vi "Sec2Timestamp.vi"(7 "Input Selection":enum32{"Time (Double)", "Time (Time Stamp)"}(radio), 10 "Input Time (Time Stamp)":timestamp format="%<%H:%M:%S%3u\n%m/%d/%y>T", 11 "Input Time (Double)":dbl format="%<%H:%M:%S>t") -> (1 "date/time string":string, 2 "Time (Time Stamp)":timestamp format="%<%H:%M:%S%3u\n%m/%d/%y>T", 3 "Time (Double)":dbl format="%<%H:%M:%S%3u\n%m/%d/%Y>T")   [LabVIEW 2018]
panel:
  out "DST (Local)":bool
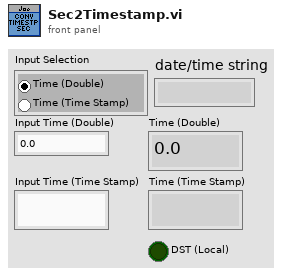
[diagram p1: front panel]
types:
  T1 = typedef "LVDateTimeRec.ctl" = cluster{"fractional second":dbl, "second":i32, "minute":i32, "hour":i32, "day of month":i32, "month":i32, "year":i32, "day of week":i32, "day of year":i32, "DST":i32}
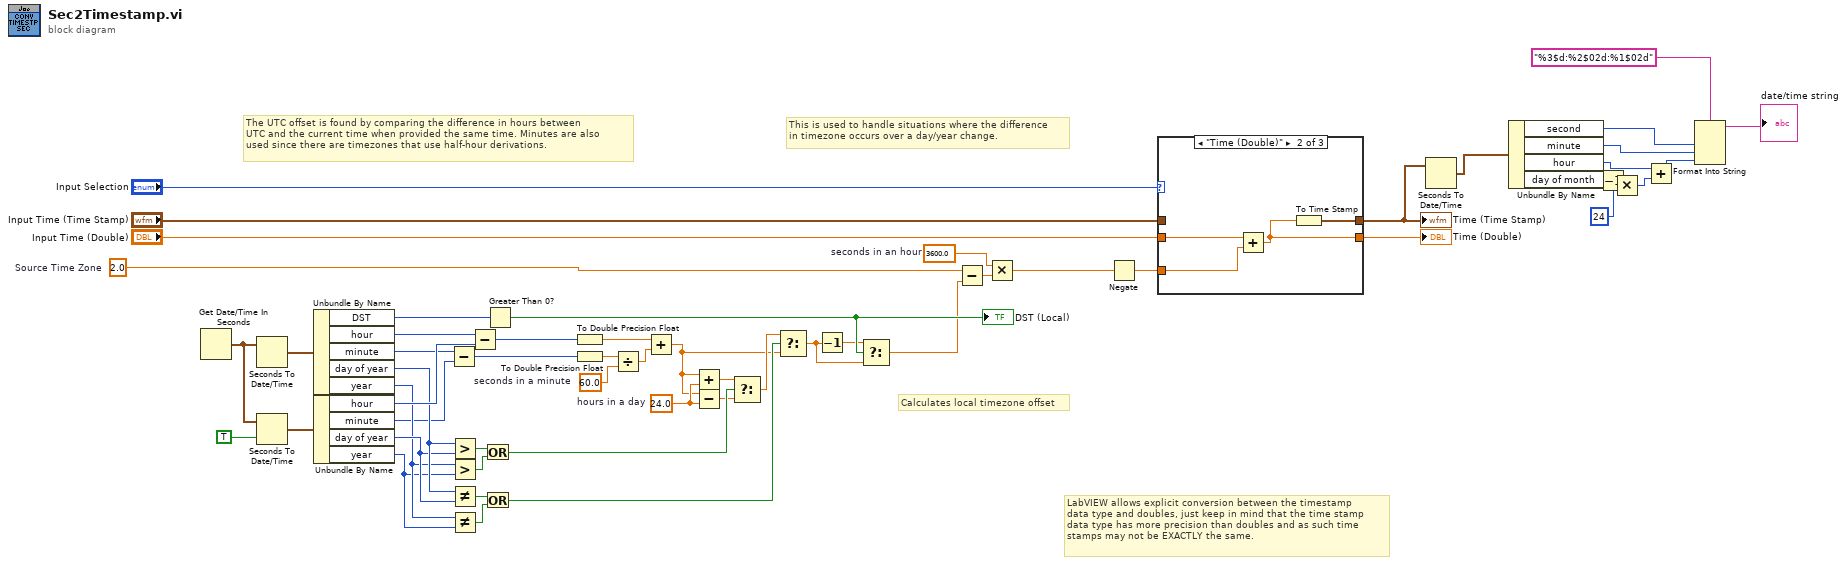
[diagram p0: block diagram]
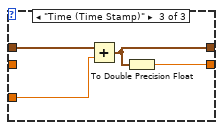
[diagram p3: hidden frame]
diagram:
  w25 = 2.0  # Source Time Zone
  w19 = 60.0  # seconds in a minute
  w34 = 24.0  # hours in a day
  w52 = 3600.0  # seconds in an hour
  # "Calculates local timezone offset"
  # "LabVIEW allows explicit conversion between the timestamp\ndata type and doubles, just keep in mind that the time stamp\ndata type has more precision than doubles and as such time\nstamps may not be EXACTLY the same."
  # "This is used to handle situations where the difference\nin timezone occurs over a day/year change."
  # "The UTC offset is found by comparing the difference in hours between\nUTC and the current time when provided the same time. Minutes are also\nused since there are timezones that use half-hour derivations."
  n1 = Get Date/Time In Seconds() -> (seconds since 1Jan1904=w49:timestamp)
  n2 = Seconds To Date/Time(time stamp (now)=w49) -> (date time rec=w46:T1)  [unwired: 1 in]
  n3 = Seconds To Date/Time(time stamp (now)=w49, to UTC (F)=TRUE) -> (date time rec=w47:T1)
  n4 = Unbundle By Name(w46) -> ("DST"=w31:i32, "hour"=w44:i32, "minute"=w22:i32, "day of year"=w41:i32, "year"=w39:i32)
  n5 = Unbundle By Name(w47) -> ("hour"=w45:i32, "minute"=w21:i32, "day of year"=w40:i32, "year"=w38:i32)
  n6 = Subtract(x=w22, y=w21) -> (x-y=w20:i32)
  n7 = Greater?(x=w41, y=w40) -> (0:w37:bool)
  n8 = Greater?(x=w39, y=w38) -> (0:w36:bool)
  n9 = Not Equal?(x=w41, y=w40) -> (x != y?=w42:bool)
  n10 = Not Equal?(x=w39, y=w38) -> (x != y?=w43:bool)
  n11 = Subtract(x=w44, y=w45) -> (x-y=w28:i32)
  n12 = Or(x=w37, y=w36) -> (x .or. y?=w35:bool)
  n13 = Or(x=w42, y=w43) -> (x .or. y?=w30:bool)
  n14 = Greater Than 0?(x=w31) -> (x > 0?=w51:bool)
  "DST (Local)" <- w51
  n15 = To Double Precision Float(number=w28) -> (double precision float=w16:dbl)
  n16 = To Double Precision Float(number=w20) -> (double precision float=w18:dbl)
  n17 = Divide(x=w18, y=w19) -> (x/y=w17:dbl)
  n18 = Add(x=w16, y=w17) -> (x+y=w15:dbl)
  n19 = Add(x=w15, y=w34) -> (x+y=w33:dbl)
  n20 = Subtract(x=w15, y=w34) -> (x-y=w32:dbl)
  n21 = Select(t=w33, s=w35, f=w32) -> (s? t:f=w29:dbl)
  n22 = Select(t=w29, s=w30, f=w15) -> (s? t:f=w27:dbl)
  n23 = Decrement(x=w27) -> (x-1=w26:dbl)
  n24 = Select(t=w26, s=w51, f=w27) -> (s? t:f=w50:dbl)
  n25 = Subtract(x=w25, y=w50) -> (x-y=w24:dbl)
  n26 = Multiply(x=w52, y=w24) -> (x*y=w23:dbl)
  n27 = Negate(x=w23) -> (-x=w14:dbl)
  n28 = case shown="\"Time (Double)\"" "Input Selection" {
    tunnel: "Input Time (Time Stamp)" -> [_ _ w63]
    tunnel: "Input Time (Double)" -> [_ w57 _]
    tunnel: w14 -> [_ w59 w62]
    tunnel: [_ w56 w60] -> w12
    tunnel: [_ w58 w61] -> w13
    frame Default {
    }
    frame "Time (Double)" {
      n29 = Add(x=w57, y=w59) -> (x+y=w58:dbl)
      n30 = To Time Stamp(1:w58) -> (0:w56:timestamp)
    }
    frame "Time (Time Stamp)" {
      n31 = Add(x=w63, y=w62) -> (x+y=w60:timestamp)
      n32 = To Double Precision Float(number=w60) -> (double precision float=w61:dbl)
    }
  }
  "Time (Double)" <- w13
  "Time (Time Stamp)" <- w12
  n33 = Seconds To Date/Time(time stamp (now)=w12) -> (date time rec=w11:T1)  [unwired: 1 in]
  n34 = Unbundle By Name(w11) -> ("second"=w10:i32, "minute"=w9:i32, "hour"=w8:i32, "day of month"=w4:i32)
  n35 = Decrement(x=w4) -> (x-1=w1:i32)
  n36 = Multiply(x=w1, y=24) -> (x*y=w2:i32)
  n37 = Add(x=w8, y=w2) -> (x+y=w7:i32)
  n38 = Format Into String(format string="%3$d:%2$02d:%1$02d", w10, w9, w7) -> (resulting string=→"date/time string":string)  [unwired: 2 in, 1 out]
